vi "Actor Core.vi"(8 "error in":errorcluster, 11 "Nested in":refnum<class "Controller.lvclass">) -> (0 "error out":errorcluster, 3 "Actor out":refnum<class "Actor.lvclass">)   [LabVIEW 2020, in "Controller.lvlib" / "Controller.lvclass"]
doc: "(<B>Filename</B>: Actor Framework.lvlib:Actor.lvclass:Actor Core.vi)\n\nReceives messages to the actor, reacts to them, and initiates any error handling that may shut the actor down.\n\nDescendant classes may override this VI to append parallel tasks for the actor to complete while it handles messages. Overrides use the Call Parent Method node."
uses:
  Controller.lvclass
  C:/Program Files (x86)/National Instruments/LabVIEW 2020/vi.lib/ActorFramework/Actor/Actor.lvclass
  <vilib>/ActorFramework/Actor/Actor.lvclass
  Coins/Coins.lvclass
  Items/Items.lvclass
  Mesage Display/Mesage Display.lvclass
  Mesage Display/Mesage Display.lvclass/Mesage Display.ctl
  Items/Items.lvclass/Items.ctl
  Coins/Coins.lvclass/Coins.ctl
  Controller.lvclass/Controller.ctl
  <vilib>/ActorFramework/Actor/Actor.lvclass/Actor.ctl
  <vilib>/ActorFramework/Message Enqueuer/Message Enqueuer.lvclass/Message Enqueuer.ctl
  <vilib>/ActorFramework/Message Enqueuer/Init from Existing Queue.vi
  <vilib>/ActorFramework/Message Enqueuer/Enqueue.vi
  <vilib>/ActorFramework/Stop Msg/Stop Msg.lvclass
  C:/Program Files (x86)/National Instruments/LabVIEW 2020/vi.lib/ActorFramework/Message/Message.lvclass
  <vilib>/ActorFramework/Message Priority Queue/Priority Enqueue.vi
  <vilib>/ActorFramework/Message Enqueuer/Message Enqueuer.lvclass
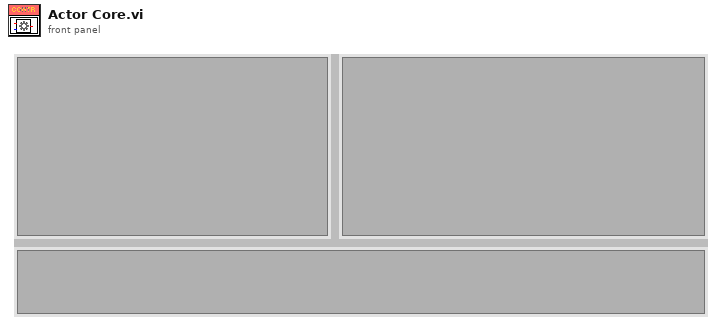
[diagram p1: front panel]
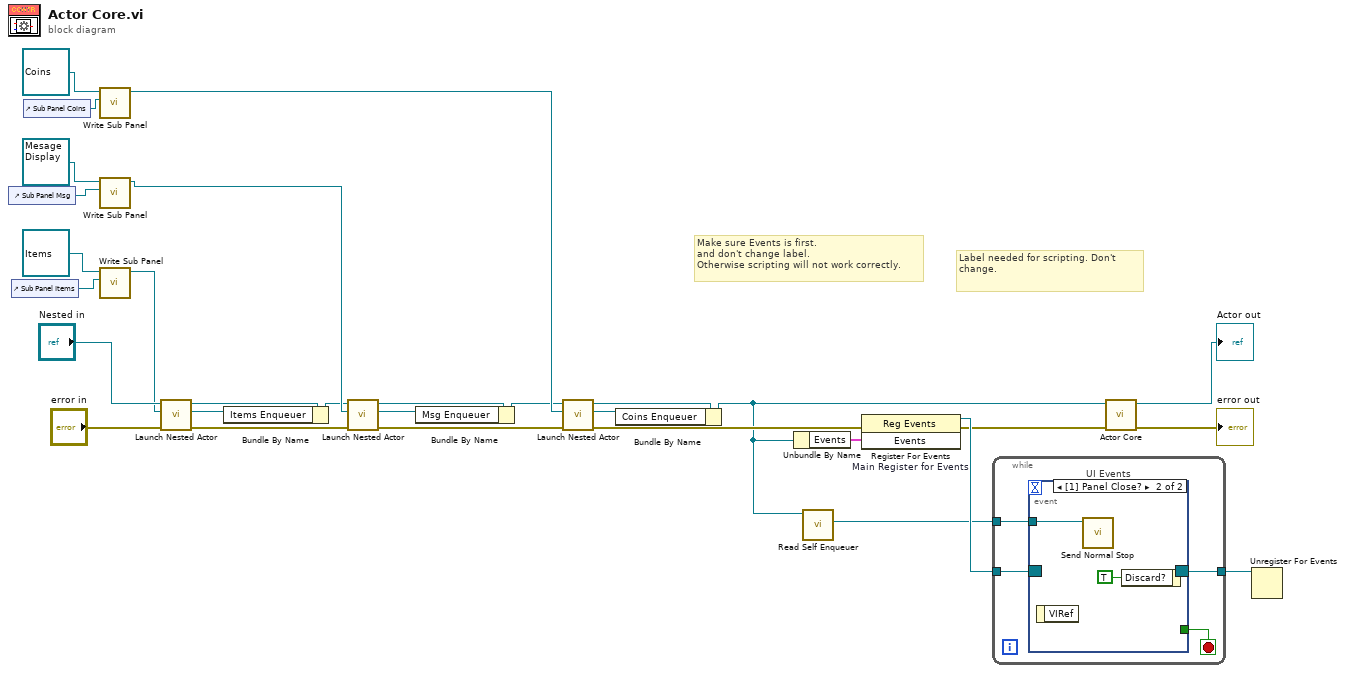
[diagram p0: block diagram]
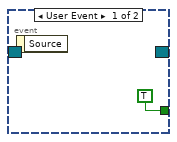
[diagram p2: hidden frame]
diagram:
  # "Label needed for scripting. Don't change."
  # "Make sure Events is first.\nand don't change label.\nOtherwise scripting will not work correctly."
  n1 = control-ref of="Sub Panel Msg"() -> (w11:refnum<vi>)
  n2 = control-ref of="Sub Panel Items"() -> (w10:refnum<vi>)
  n3 = control-ref of="Sub Panel Coins"() -> (w12:refnum<vi>)
  n4 = call "Write Sub Panel.vi"("Sub Panel"=w12, "Coins in"=refnum<class "Coins.lvclass"> refnum ("Coins.lvlib:Coins.lvclass")) -> ("Coins out"=w7:refnum<class "Coins.lvclass">)  [unwired: 8 in, 1 out]
  n5 = call "Write Sub Panel.vi"("Sub Panel"=w11, "Mesage Display in"=refnum<class "Mesage Display.lvclass"> refnum ("Mesage Display.lvlib:Mesage Display.lvclass")) -> ("Mesage Display out"=w8:refnum<class "Mesage Display.lvclass">)  [unwired: 8 in, 1 out]
  n6 = call "Write Sub Panel.vi"("Sub Panel"=w10, "Items in"=refnum<class "Items.lvclass"> refnum ("Items.lvlib:Items.lvclass")) -> ("Items out"=w9:refnum<class "Items.lvclass">)  [unwired: 8 in, 1 out]
  n7 = call <vilib>:"Launch Nested Actor.vi"("error in (no error)"="error in", "Nested Actor"=w9, "Caller Actor in"="Nested in") -> ("error out"=w18:errorcluster, "Nested Actor's Enqueuer"=w5:refnum<class "Message Enqueuer.lvclass">, "Caller Actor out"=w16:refnum<class "Controller.lvclass">)  [unwired: 6 in]
  n8 = Bundle By Name(cluster=w16, "Items Enqueuer"=w5) -> (w6:refnum<class "Controller.lvclass">)
  n9 = call <vilib>:"Launch Nested Actor.vi"("error in (no error)"=w18, "Nested Actor"=w8, "Caller Actor in"=w6) -> ("error out"=w20:errorcluster, "Nested Actor's Enqueuer"=w3:refnum<class "Message Enqueuer.lvclass">, "Caller Actor out"=w19:refnum<class "Controller.lvclass">)  [unwired: 6 in]
  n10 = Bundle By Name(cluster=w19, "Msg Enqueuer"=w3) -> (w4:refnum<class "Controller.lvclass">)
  n11 = call <vilib>:"Launch Nested Actor.vi"("error in (no error)"=w20, "Nested Actor"=w7, "Caller Actor in"=w4) -> ("error out"=w22:errorcluster, "Nested Actor's Enqueuer"=w1:refnum<class "Message Enqueuer.lvclass">, "Caller Actor out"=w21:refnum<class "Controller.lvclass">)  [unwired: 6 in]
  n12 = Bundle By Name(cluster=w21, "Coins Enqueuer"=w1) -> (w2:refnum<class "Controller.lvclass">)
  n13 = Unbundle By Name(w2) -> ("Events"=w23:cluster{"Stop":refnum<user-event>})
  n14 = call <vilib>:"Read Self Enqueuer.vi"("Actor"=w2) -> ("Self Enqueuer"=w26:refnum<class "Message Enqueuer.lvclass">)  [unwired: 10 in]
  n15 = register-events "Main Register for Events"(error in=w22, w23) -> (reference out=w28:refnum<event-registration>, error out=w24:errorcluster)  [unwired: 1 in]
  n16 = while {
    tunnel: w28 -> [w34]
    tunnel: [w32] -> w27
    tunnel: w26 -> [w31]
    stop <- w33 stop-if-true
    n17 = event "UI Events" shown="[1] Panel Close?" {
      selector: w34 -> [_ _]
      dyn-events: [_ _] -> w32
      timeout: _ -> [_ _]
      tunnel: [TRUE _] -> w33
      tunnel: w31 -> [_ w36]
      event User Event {
        n18 = event-data() -> ()  [unwired: 1 in, 1 out]
      }
      event Panel Close? {
        n19 = event-data() -> ()  [unwired: 1 in, 1 out]
        n20 = call <vilib>:"Send Normal Stop.vi"("Message Enqueuer"=w36) -> ()  [unwired: 10 in, 1 out]
        n21 = event-data("Discard?"=TRUE) -> ()  [unwired: 1 in, 1 out]
      }
    }
  }
  n22 = call-parent "Actor Core.vi"("error in"=w24, "Actor in"=w2) -> ("error out"=→"error out":errorcluster, "Actor out"=→"Actor out":refnum<class "Actor.lvclass">)  [unwired: 8 in]
  n23 = Unregister For Events(event registration refnum=w27) -> ()  [unwired: 1 in, 1 out]
